vi "error_handler.vi"(6 "Additional info":string, 8 "error in (no error)":errorcluster, 9 "name of caller in (you)":string, 10 "code (0 = no error)":i32) -> (0 "error out":errorcluster, 1 "error in self?":bool)   [LabVIEW 2015]
uses:
  poly_global_eco_plus.vi
  _error_tools_polys.lvlib
panel:
  # "ECO = Error Code Offset"
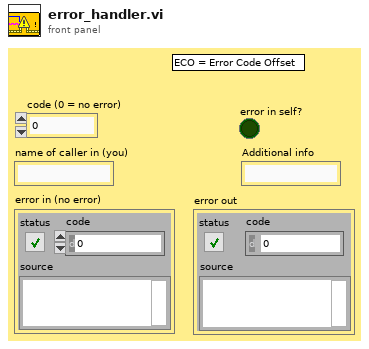
[diagram p1: front panel]
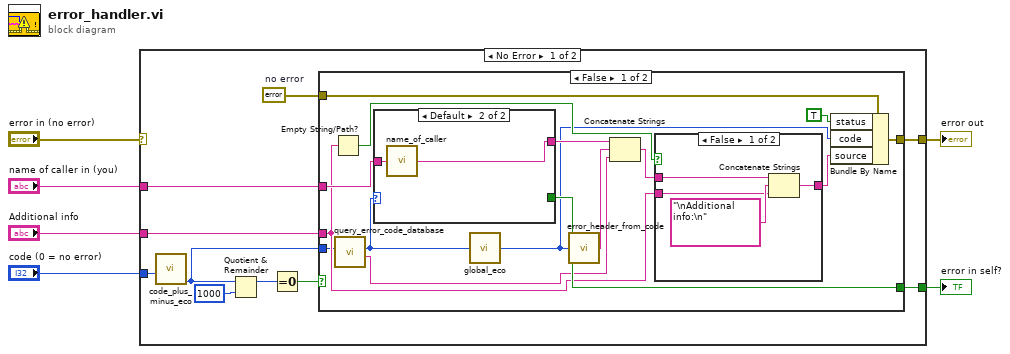
[diagram p0: block diagram]
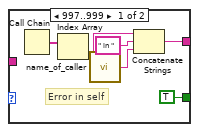
[diagram p3: hidden frame]
diagram:
  n1 = case shown="No Error" "error in (no error)" {
    selector: "error in (no error)" -> [_ w46]
    tunnel: "name of caller in (you)" -> [w15 _]
    tunnel: "code (0 = no error)" -> [w10 _]
    tunnel: [w13 _] -> w4
    tunnel: [w12 w46] -> w2
    tunnel: "Additional info" -> [w11 _]
    frame No Error {
      w16 = errorcluster {"status"=FALSE, "code"=0, "source"=""}  # no error
      n2 = call "code_plus_minus_eco.vi"("code in"=w10) -> ("code w/out ECO"=w9:i32)  [unwired: 9 in, 1 out]
      n3 = Quotient & Remainder(x=w9, y=1000) -> (x-y*floor(x/y)=w7:i32)  [unwired: 1 out]
      n4 = Equal To 0?(x=w7) -> (x = 0?=w14:bool)
      n5 = case shown="False" w14 {
        tunnel: w16 -> [w31 w45]
        tunnel: [w30 w45] -> w12
        tunnel: w9 -> [w19 _]
        tunnel: w15 -> [w29 _]
        tunnel: [w26 _] -> w13
        tunnel: w11 -> [w22 _]
        frame False {
          n6 = Empty String/Path?(string/path=w22) -> (empty?=w25:bool)
          n7 = call "query_error_code_database.vi"("code in"=w19) -> ("code description"=w17:string, "code out"=w18:i32)  [unwired: 9 in]
          n8 = case shown="Default" w18 {
            tunnel: w29 -> [_ w44]
            tunnel: [w38 w43] -> w28
            tunnel: [TRUE _] -> w26
            frame 997..999 {
              # "Error in self"
              # "Error in this vi"
              n9 = Call Chain() -> (call chain=w42:string[])
              n10 = Index Array(array=w42) -> (element=w41:string)  [unwired: 1 in]
              n11 = call "name_of_caller.vi"() -> ("name of caller out"=w39:string)  [unwired: 4 in]
              n12 = Concatenate Strings(w41, " in " ("string"), w39) -> (w38:string)
            }
            frame Default {
              n13 = call "name_of_caller.vi"("name of caller in"=w44) -> ("name of caller out"=w43:string)  [unwired: 3 in]
            }
          }
          n14 = call-poly "global_eco.vi"("code (w/out ECO)"=w18) -> ("code (+ ECO)"=w21:i32)  [unwired: 4 in]
          n15 = call "error_header_from_code.vi"("Error/warning code"=w21) -> ("error_header"=w20:string)  [unwired: 4 in]
          n16 = Concatenate Strings(w28, w20, w17) -> (w24:string)
          n17 = case shown="False" w25 {
            tunnel: w24 -> [w35 w36]
            tunnel: [w32 w36] -> w23
            tunnel: w22 -> [w33 _]
            frame False {
              n18 = Concatenate Strings(w35, "\nAdditional info:\n" ("string"), w33) -> (w32:string)
            }
            frame True {
            }
          }
          n19 = Bundle By Name(cluster=w31, "status"=TRUE, "code"=w21, "source"=w23) -> (w30:errorcluster)
        }
        frame True {
        }
      }
    }
    frame Error {
    }
  }
  "error out" <- w2
  "error in self?" <- w4
